vi "H1_H2.vi"(8 "H2 MSB":u8, 9 "H2 LSB":u8, 10 "H1 MSB":u8, 11 "H1 LSB":u8) -> (1 "H2":u16, 2 "H1":u16)   [LabVIEW 2022 SP3, in "BME680.lvlib" / "BME680.lvclass"]
uses:
  BME680.lvclass
  BME680.lvclass/BME680.ctl
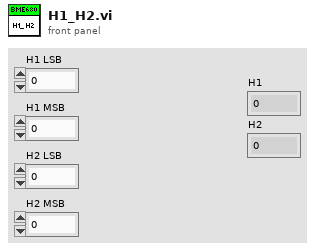
[diagram p1: front panel]
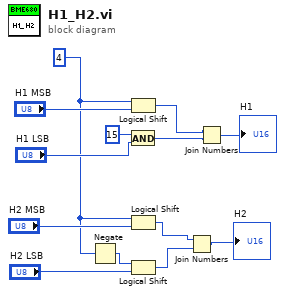
[diagram p0: block diagram]
diagram:
  w7 = i16 4 ("y")
  n1 = Negate(x=w7) -> (-x=w8:i16)
  n2 = Logical Shift(y=w7, x="H1 MSB") -> (x << y=w5:u8)
  n3 = And(x=u8 15, y="H1 LSB") -> (x .and. y?=w6:u8)
  n4 = Logical Shift(y=w7, x="H2 MSB") -> (x << y=w2:u8)
  n5 = Logical Shift(y=w8, x="H2 LSB") -> (x << y=w3:u8)
  n6 = Join Numbers(hi=w2, lo=w3) -> ((hi.lo)=→"H2":u16)
  n7 = Join Numbers(hi=w5, lo=w6) -> ((hi.lo)=→"H1":u16)
